vi "get_params.vi"(8 "error in (no error)":errorcluster caption="entrée d'erreur (pas d'erreur)", 11 "MeanShift.lvclass 2":refnum<class "MeanShift.lvclass">) -> (0 "error out":errorcluster caption="sortie d'erreur", 3 "MeanShift.lvclass":refnum<class "MeanShift.lvclass">)   [LabVIEW 2020, in "MeanShift.lvclass"]
uses:
  MeanShift.lvclass
  MeanShift.lvclass/MeanShift.ctl
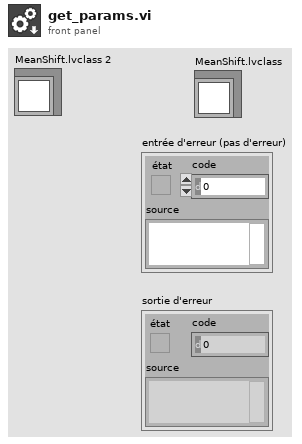
[diagram p1: front panel]
types:
  T1 = typedef "mean_shift_params.ctl" = cluster{"bandwidth":cluster{"bandwidth_type":string, "bandwidth_float":dbl}, "seeds":cluster{"seeds_type":string, "seeds_list":dbl[][]}, "bin_seeding":bool, "min_bin_freq":dbl, "cluster_all":bool, "n_jobs":dbl, "max_iter":dbl}
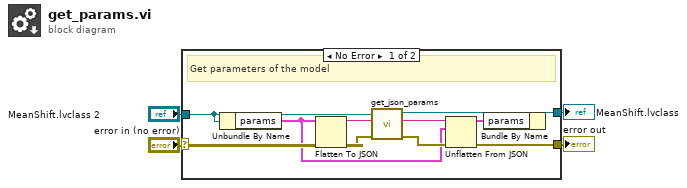
[diagram p0: block diagram]
diagram:
  n1 = case shown="No Error" "error in (no error)" {
    selector: "error in (no error)" -> [w13 w16]
    tunnel: [w5 w16] -> w3
    tunnel: "MeanShift.lvclass 2" -> [w10 w17]
    tunnel: [w7 w17] -> w1
    frame No Error {
      # "Get parameters of the model"
      n2 = Unbundle By Name(w10) -> ("params"=w9:T1)
      n3 = Flatten To JSON(anything=w9, error in (no error)=w13) -> (JSON string=w12:string, 11:w11:errorcluster)  [unwired: 1 in]
      n4 = call-dynamic "get_json_params.vi"("error in (no error)"=w11, "format"=w12, "Model en entrée"=w10) -> ("error out"=w14:errorcluster, "valeur renvoyée"=w15:string, "Model en sortie"=w8:refnum<class "MeanShift.lvclass">)  [unwired: 6 in]
      n5 = Unflatten From JSON(JSON string=w15, type and defaults=w9, error in (no error)=w14) -> (value=w6:T1, error out=w5:errorcluster)  [unwired: 4 in]
      n6 = Bundle By Name(cluster=w8, "params"=w6) -> (w7:refnum<class "MeanShift.lvclass">)
    }
    frame Error {
    }
  }
  "error out" <- w3
  "MeanShift.lvclass" <- w1
